vi "Array Functions Activity.vi"() -> ()   [LabVIEW 2014]
panel:
  out "Deleted portion":dbl[][](array[numeric])
  out "Output Array":dbl[][](array[numeric])
  out "Output Array":dbl[][](array[numeric])
  out "Index of Element":i32
  out "2D Array (Integer)":i32[][](array[numeric])
  out "1D Array (DBL)":dbl[](array[numeric])
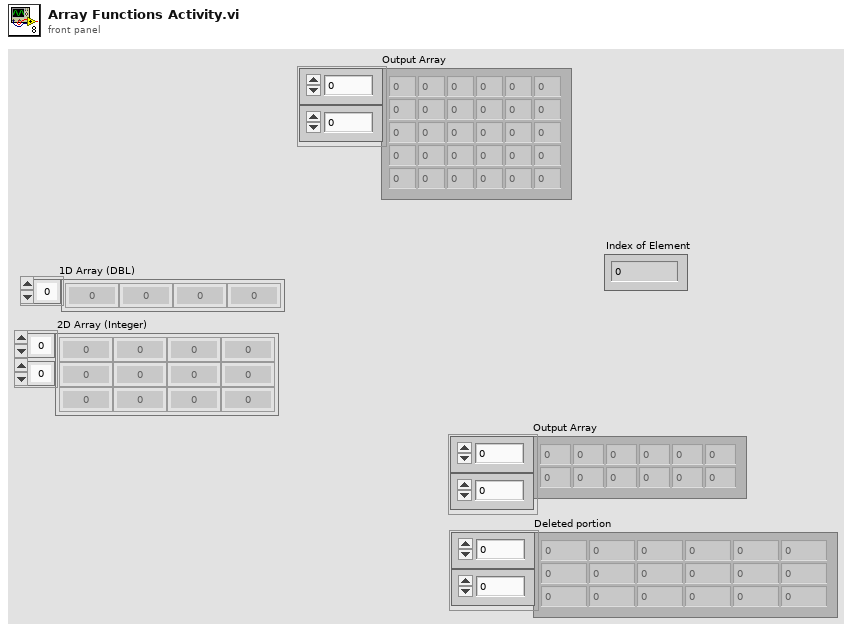
[diagram p1: front panel]
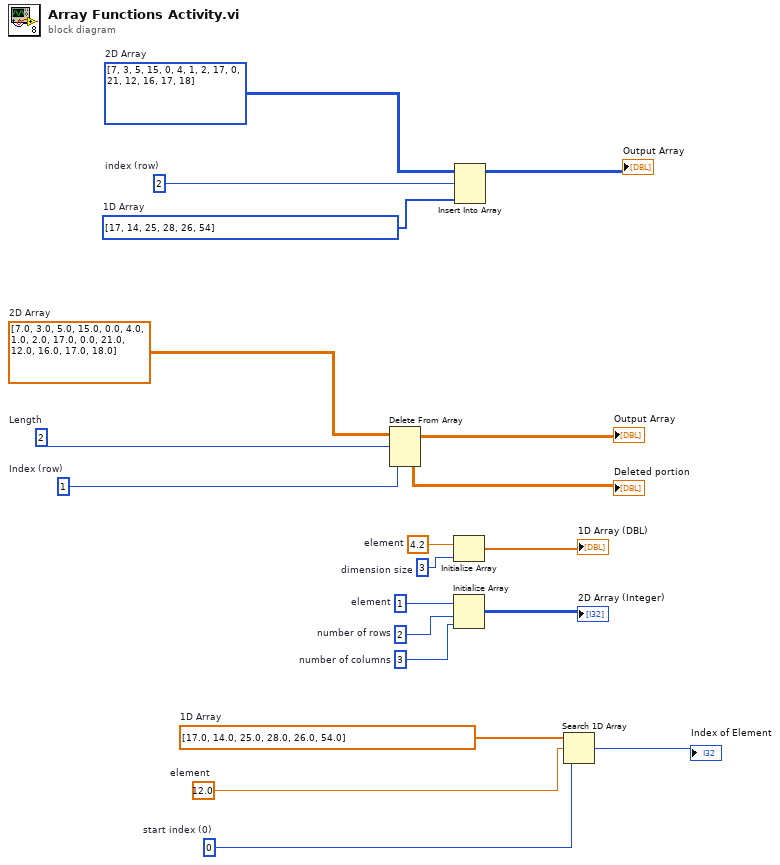
[diagram p0: block diagram]
diagram:
  w3 = 1  # Index (row)
  w4 = 2  # Length
  w5 = dbl[][] [[7.0, 3.0, 5.0, 15.0, 0.0], [4.0, 1.0, 2.0, 17.0, 0.0], [21.0, 12.0, 16.0, 17.0, 18.0]]  # 2D Array
  w7 = i32[] [17, 14, 25, 28, 26, 54]  # 1D Array
  w8 = 2  # index (row)
  w11 = 0  # start index (0)
  w12 = 12.0  # element
  w13 = dbl[] [17.0, 14.0, 25.0, 28.0, 26.0, 54.0]  # 1D Array
  w15 = 3  # number of columns
  w16 = 2  # number of rows
  w17 = 1  # element
  w19 = 3  # dimension size
  w20 = 4.2  # element
  w9 = i32[][] [[7, 3, 5, 15, 0], [4, 1, 2, 17, 0], [21, 12, 16, 17, 18]]  # 2D Array
  n1 = Delete From Array "Delete From Array"(array=w5, length=w4, index (row)=w3) -> (deleted portion=→"Deleted portion":dbl[][], array with subset deleted=→"Output Array":dbl[][])  [unwired: 1 in]
  n2 = Initialize Array "Initialize Array"(w20, w19) -> (→"1D Array (DBL)":dbl[])
  n3 = Initialize Array "Initialize Array"(w17, w16, w15) -> (→"2D Array (Integer)":i32[][])
  n4 = Insert Into Array "Insert Into Array"(array=w9, index (row)=w8, new element=w7) -> (→"Output Array":i32[][])  [unwired: 1 in]
  n5 = Search 1D Array(1D array=w13, element=w12, start index (0)=w11) -> (index of element=→"Index of Element":i32)
